vi "Sample_and_Hold.vi"(1 "Sample or Hold?":bool, 2 "Input":dbl) -> (0 "Output":dbl)   [LabVIEW 2016]
doc: "Help by FRC Team 836 - The RoboBees\n\nThis VI will either continually display new input values when set \"Sample\" or hold the current value when set to \"Hold\"."
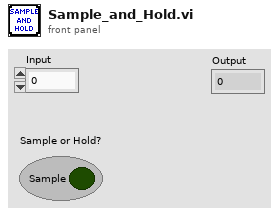
[diagram p1: front panel]
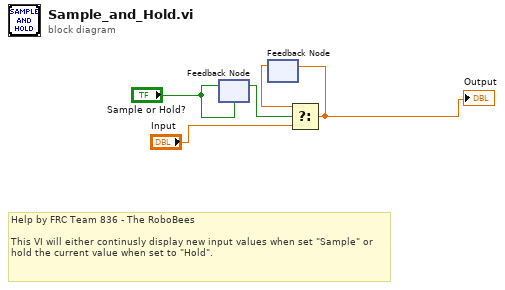
[diagram p0: block diagram]
diagram:
  # "Help by FRC Team 836 - The RoboBees\n\nThis VI will either continusly display new input values when set \"Sample\" or hold the current value when set to \"Hold\"."
  n1 = feedback #1("Sample or Hold?") -> (w1:bool)
  n2 = feedback-in #1("Sample or Hold?") -> ()
  n3 = feedback #2() -> (w4:dbl)  [unwired: 1 in]
  n4 = Select(t=w4, s=w1, f="Input") -> (s? t:f=w3:dbl)
  "Output" <- w3
  n5 = feedback-in #2(w3) -> ()
